vi "Probe.vi"(11 "Gen2":refnum<class "KDemoDerived.lvclass">) -> (2 "Value String":string, 3 "Boolean":bool)   [LabVIEW 2015]
uses:
  KDemoDerived.lvclass
  KDemoDerived.lvclass/KDemoDerived.ctl
panel:
  out "Integer":i32
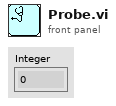
[diagram p1: front panel]
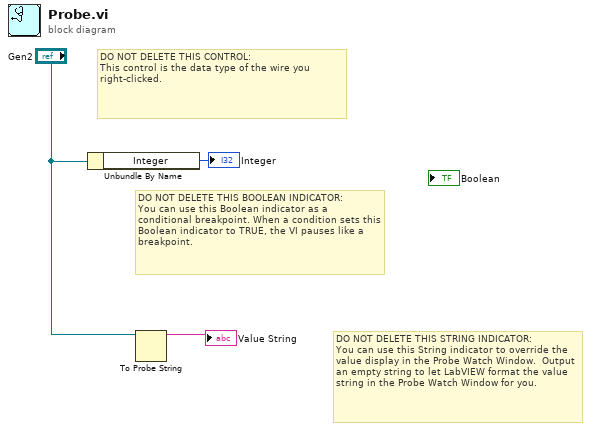
[diagram p0: block diagram]
diagram:
  # "DO NOT DELETE THIS STRING INDICATOR: \nYou can use this String indicator to override the value display in the Probe Watch Window.  Output an empty string to let LabVIEW format the value string in the Probe Watch Window for you."
  # "DO NOT DELETE THIS BOOLEAN INDICATOR: \nYou can use this Boolean indicator as a conditional breakpoint. When a condition sets this Boolean indicator to TRUE, the VI pauses like a breakpoint."
  # "DO NOT DELETE THIS CONTROL: \nThis control is the data type of the wire you right-clicked."
  n1 = Unbundle By Name("Gen2") -> ("Integer"=→"Integer":i32)
  n2 = To Probe String(7:"Gen2") -> (3:→"Value String":string)  [unwired: 2 in, 1 out]
